vi "Calculate Nominal Resistance.vi"(8 "error in (no error)":errorcluster, 9 "Number of Bands":T3=4 min=3 max=6 step=1, 10 "M sel":T4, 11 "Resistance Digits":T1) -> (0 "error out":errorcluster, 3 "Nominal Value":dbl format="%#_2p")   [LabVIEW 2018, in "Resistance Value.lvlib"]
doc: "Calculates the nominal resistance value from the resistor band selections and number of bands.\n\nThe VI receives the <b>Number of Bands</b>, the <b>1D sel</b>, <b>2D sel</b>, <b>3D sel</b>, and <b>M sel</b> inputs and returns the calculated <b>Nominal</b> resistance value."
uses:
  Resistance Value.lvlib
  Mmultiplier--enum.ctl
  Number of Bands--number.ctl
  Resistance Digits--cluster.ctl
  Ddigit--enum.ctl
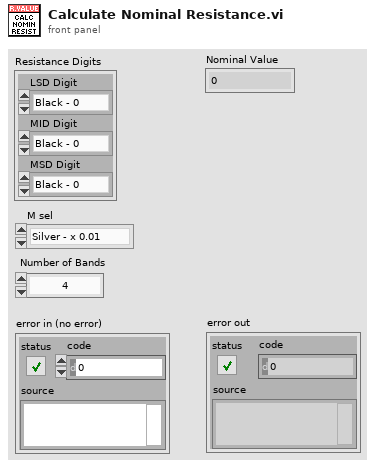
[diagram p1: front panel]
types:
  T1 = typedef "Resistance Digits--cluster.ctl" = cluster{"LSD Digit":T2, "MID Digit":T2, "MSD Digit":T2}
  T2 = typedef "Ddigit--enum.ctl" = enum16{"Black - 0", "Brown - 1", "Red - 2", "Orange - 3", "Yellow - 4", "Green - 5", "Blue - 6", "Violet - 7", "Grey - 8", "White - 9"}
  T3 = typedef "Number of Bands--number.ctl" = u8
  T4 = typedef "Mmultiplier--enum.ctl" = enum16{"Silver - x 0.01", "Gold - x 0.1 ", "Black - x 1", "Brown - x 10", "Red - x 100", "Orange - x 1k", "Yellow - x 10k", "Green - 100k", "Blue - x 1M", "Violet - x10 M", "Grey - x 100M", "White - x 1G"}
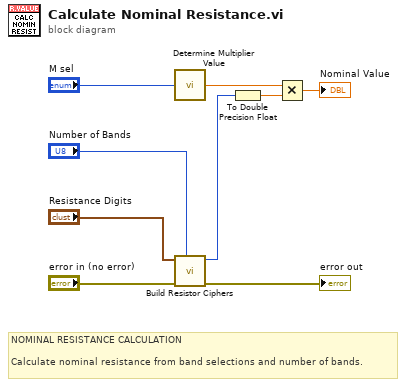
[diagram p0: block diagram]
diagram:
  # "NOMINAL RESISTANCE CALCULATION\n\nCalculate nominal resistance from band selections and number of bands."
  n1 = call "Determine Multiplier Value.vi"("mult color"="M sel") -> ("multiplier"=w5:dbl)  [unwired: 6 in]
  n2 = call "Build Resistor Ciphers.vi"("Number of Bands"="Number of Bands", "error in (no error)"="error in (no error)", "Resistance Digits"="Resistance Digits") -> ("error out"=→"error out":errorcluster, "Nominal Value"=w4:i32)  [unwired: 6 in, 1 out]
  n3 = To Double Precision Float(number=w4) -> (double precision float=w6:dbl)
  n4 = Multiply(x=w5, y=w6) -> (x*y=→"Nominal Value":dbl)
